vi "Read Bandwidth (nm).vi"(8 "error in (no error)":errorcluster, 11 "Light Source in":refnum<class "Light Source.lvclass">) -> (0 "error out":errorcluster, 2 "Bandwidth (nm)":dbl, 3 "Light Source out":refnum<class "Light Source.lvclass">)   [LabVIEW 2017, in "Light Source.lvclass"]
uses:
  Light Source.lvclass
  Light Source.lvclass/Light Source.ctl
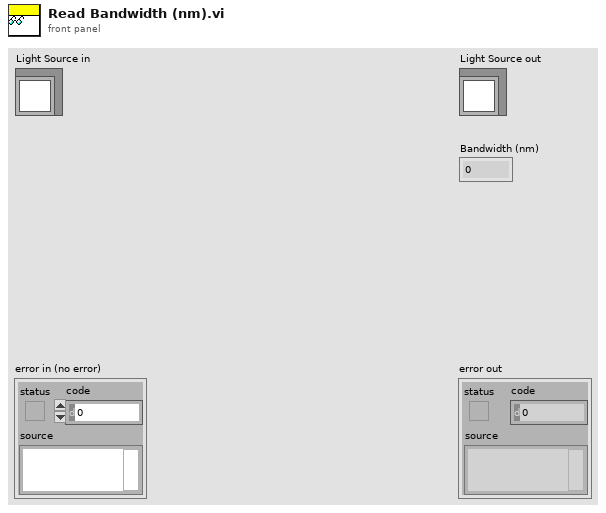
[diagram p1: front panel]
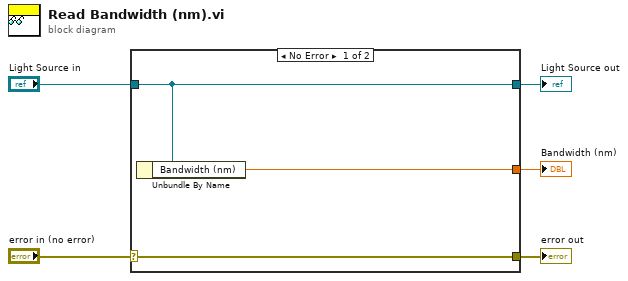
[diagram p0: block diagram]
diagram:
  n1 = case shown="No Error" "error in (no error)" {
    selector: "error in (no error)" -> [w8 w9]
    tunnel: [w8 w9] -> w4
    tunnel: [w7 w10] -> w2
    tunnel: "Light Source in" -> [w7 w10]
    tunnel: [w6 _] -> w1
    frame No Error {
      n2 = Unbundle By Name(w7) -> ("Bandwidth (nm)"=w6:dbl)
    }
    frame Error {
    }
  }
  "error out" <- w4
  "Light Source out" <- w2
  "Bandwidth (nm)" <- w1
